vi "fgt get power.vi"(8 "error in (no error)":errorcluster, 11 "controllerIndex":u16) -> (0 "error out":errorcluster, 3 "powerState":T1)   [LabVIEW 2016, in "fgt_SDK.lvlib"]
doc: "Get power information about a controller (such as Link, MFCS, Flowboard).\nNot all controllers support this functionality."
uses:
  fgt_SDK.lvlib
  TypeDefs/fgt_POWER.ctl
  dlls/fgt_SDK_32.dll
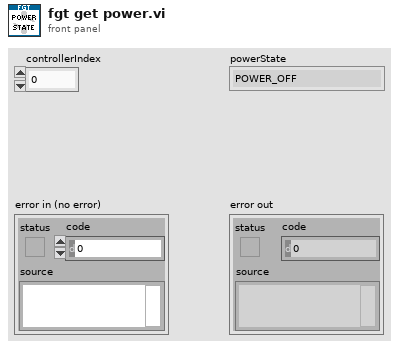
[diagram p1: front panel]
types:
  T1 = typedef "fgt_SDK.lvlib/fgt_POWER.ctl" = enum8{"POWER_OFF", "POWER_ON", "SLEEP"}
  T2 = typedef "fgt_SDK.lvlib/fgt_STATUS_INFO.ctl" = cluster{"InstrType":T3, "instrSN":u16, "errorCode":u8, "infoCode":u8, "detail":string}
  T3 = typedef "fgt_SDK.lvlib/fgt_INSTRUMENT_TYPE.ctl" = enum32{"None", "MFCS", "MFCS_EZ", "FRP", "LineUP", "IPS"}
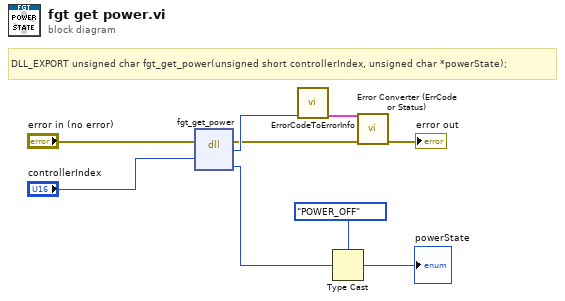
[diagram p0: block diagram]
diagram:
  # "DLL_EXPORT unsigned char fgt_get_power(unsigned short controllerIndex, unsigned char *powerState);"
  n1 = dll-call lib="C:/projects/SDK/fgt-sdk-labview/dlls/fgt_SDK_*.*" fn="fgt_get_power"(error in="error in (no error)", "controllerIndex"="controllerIndex") -> (error out=w4:errorcluster, "return type"=w6:u8, "powerState"=w1:u8)  [unwired: 4 in, 1 out]
  n2 = call "ErrorCodeToErrorInfo.vi"("return type"=w6) -> ("StatusInfo"=w5:T2)  [unwired: 10 in]
  n3 = Type Cast(type=fgt_POWER."POWER_OFF" ("powerState"), x=w1) -> (*(type *) &x=→"powerState":T1)
  n4 = call "Error Converter (ErrCode or Status).vi"("error in (no error)"=w4, "StatusInfo"=w5) -> ("error out"=→"error out":errorcluster)  [unwired: 9 in]
